vi "Update Combo Box Control Value By Name.vi"(6 "Disabled":T1(ring), 7 "Strings []":string[](array[string]), 8 "error in (no error)":errorcluster, 9 "Data":string, 10 "Combo Box Control Name":string, 11 "Controls[]":refnum<vi>[](array[refnum])) -> (0 "error out":errorcluster, 3 "Controls[] Out":refnum<vi>[](array[refnum]))   [LabVIEW 2021]
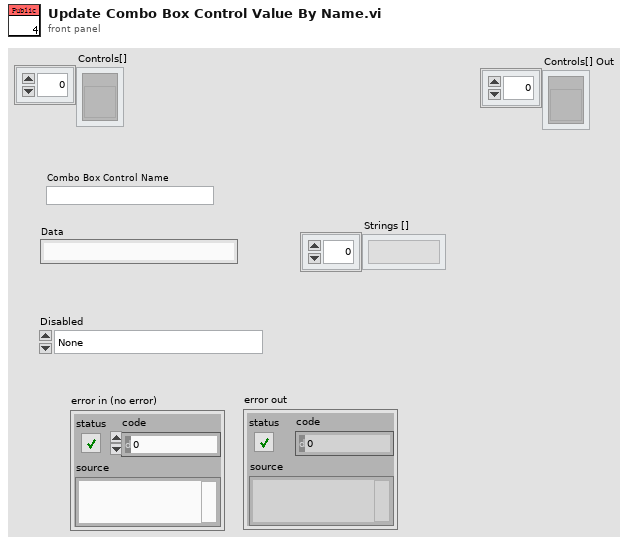
[diagram p1: front panel]
types:
  T1 = enum8{"None", "Enabled", "Disabled", "Disabled and Grayed Out", ""}
  T2 = enum8{"Enabled", "Disabled", "Disabled and Grayed Out"}
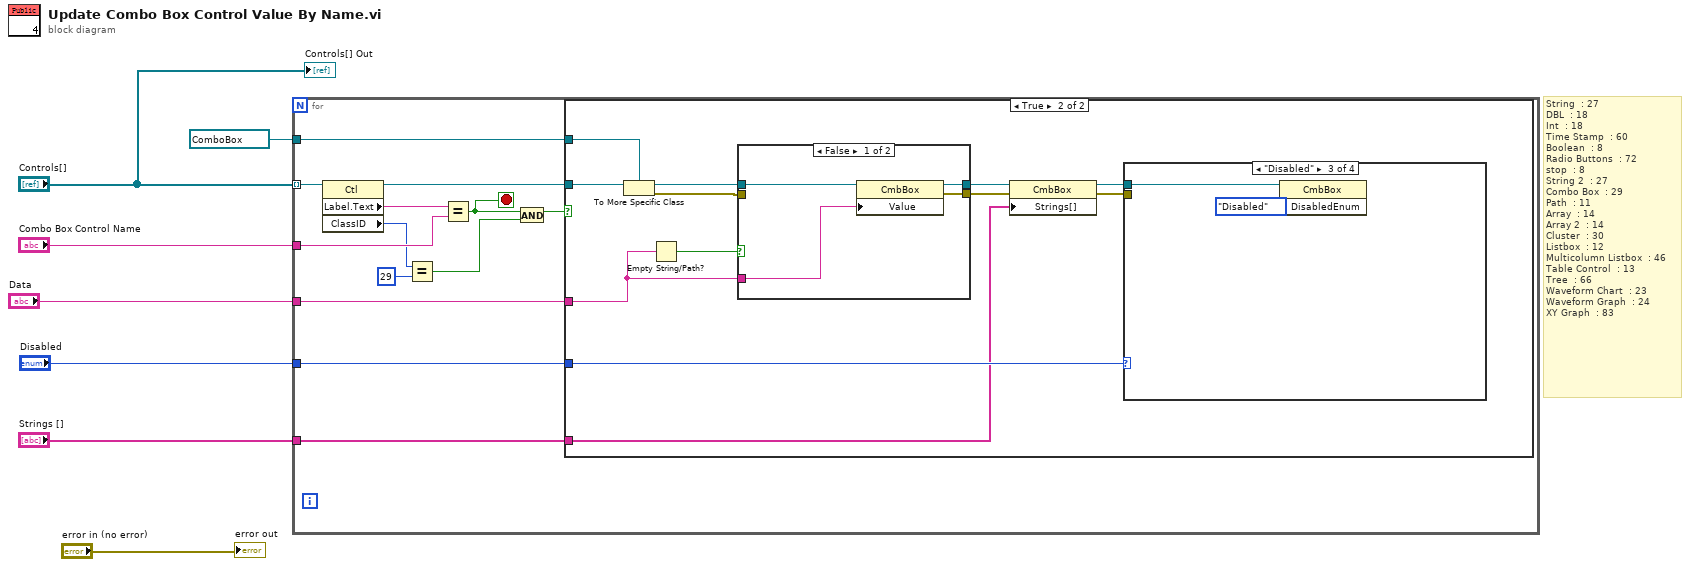
[diagram p0: block diagram]
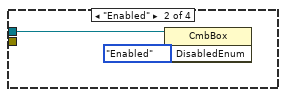
[diagram p5: hidden frame]
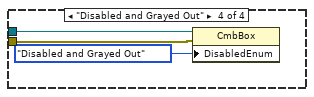
[diagram p6: hidden frame]
diagram:
  # "String  : 27\nDBL  : 18\nInt  : 18\nTime Stamp  : 60\nBoolean  : 8\nRadio Buttons  : 72\nstop  : 8\nString 2  : 27\nCombo Box  : 29\nPath  : 11\nArray  : 14\nArray 2  : 14\nCluster  : 30\nListbox  : 12\nMulticolumn Listbox  : 46\nTable Control  : 13\nTree  : 66\nWaveform Chart  : 23\nWaveform Graph  : 24\nXY Graph  : 83"
  n1 = for {
    tunnel: "Controls[]" -> [w20] mode=indexing
    tunnel: "Combo Box Control Name" -> [w18]
    tunnel: "Data" -> [w15]
    tunnel: "Disabled" -> [w14]
    tunnel: refnum<vi> refnum ("Combo Box") -> [w13]
    tunnel: "Strings []" -> [w8]
    stop <- w17 stop-if-true
    n2 = property class="Ctl"(reference=w20) -> (reference out=w16:refnum<vi>, "Label.Text"=w19:string, "ClassID"=w12:u32)  [unwired: 1 in, 1 out]
    n3 = Equal?(x=w12, y=u32 29) -> (x = y?=w9:bool)
    n4 = Equal?(x=w19, y=w18) -> (x = y?=w17:bool)
    n5 = And(x=w17, y=w9) -> (x .and. y?=w10:bool)
    n6 = case shown="True" w10 {
      tunnel: w16 -> [_ w31]
      tunnel: w15 -> [_ w23]
      tunnel: w14 -> [_ w30]
      tunnel: w13 -> [_ w29]
      tunnel: w8 -> [_ w24]
      frame False {
      }
      frame True {
        n7 = To More Specific Class(target class=w29, reference=w31) -> (specific class reference=w32:refnum<vi>, error out=w21:errorcluster)  [unwired: 1 in]
        n8 = Empty String/Path?(string/path=w23) -> (empty?=w22:bool)
        n9 = case shown="False" w22 {
          tunnel: w32 -> [w36 w38]
          tunnel: [w35 w38] -> w28
          tunnel: [w34 w37] -> w26
          tunnel: w23 -> [w33 _]
          tunnel: w21 -> [_ w37]
          frame False {
            n10 = property class="CmbBox"(reference=w36, "Value"=w33) -> (reference out=w35:refnum<vi>, error out=w34:errorcluster)  [unwired: 1 in]
          }
          frame True {
          }
        }
        n11 = property class="CmbBox"(reference=w28, error in=w26, "Strings[]"=w24) -> (reference out=w27:refnum<vi>, error out=w25:errorcluster)
        n12 = case shown="\"Disabled\"" w30 {
          tunnel: w27 -> [_ w40 w42 w45]
          tunnel: w25 -> [_ _ _ w43]
          frame "None", Default {
          }
          frame "Enabled" {
            n13 = property class="CmbBox"(reference=w40, "DisabledEnum"=T2."Enabled" ("Disabled")) -> ()  [unwired: 1 in, 2 out]
          }
          frame "Disabled" {
            n14 = property class="CmbBox"(reference=w42, "DisabledEnum"=T2."Disabled" ("Disabled")) -> ()  [unwired: 1 in, 2 out]
          }
          frame "Disabled and Grayed Out" {
            n15 = property class="CmbBox"(reference=w45, error in=w43, "DisabledEnum"=T2."Disabled and Grayed Out" ("Disabled")) -> ()  [unwired: 2 out]
          }
        }
      }
    }
  }
  "error out" <- "error in (no error)"
  "Controls[] Out" <- "Controls[]"
